vi "Set State.vi"(8 "error in (no error)":errorcluster, 10 "Device State":T1, 11 "Device in":refnum<class "Device.lvclass">) -> (0 "error out":errorcluster, 3 "Device out":refnum<class "Device.lvclass">)   [LabVIEW 2020, in "HAL.lvlib" / "Device.lvclass"]
uses:
  Device.lvclass
  Device State.ctl
  Device.lvclass/Device.ctl
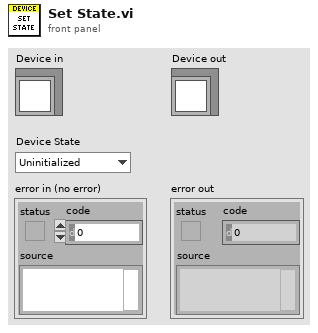
[diagram p1: front panel]
types:
  T1 = typedef "HAL.lvlib/Device.lvclass/Device State.ctl" = enum16{"Uninitialized", "Initialized", "Running", "Error"}
  T2 = typedef "HAL.lvlib/Device.lvclass/Ref Data.ctl" = cluster{"Config Keys":string[], "Config Values":string[], "Cal Expires":timestamp, "Name":string, "Comment":string, "State":T1, "Error":errorcluster}
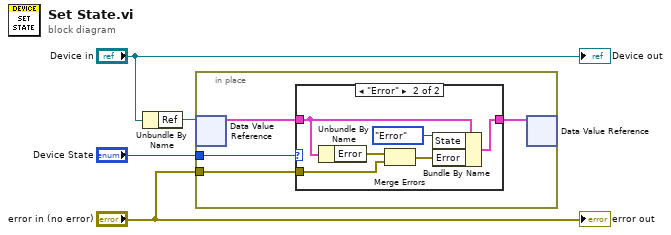
[diagram p0: block diagram]
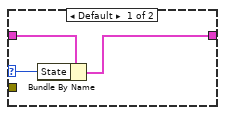
[diagram p2: hidden frame]
diagram:
  n1 = Unbundle By Name("Device in") -> ("Ref"=w4:refnum<data-value>)
  n2 = in-place {
    in-place-border: "Device State" -> [w8]
    in-place-border: "error in (no error)" -> [w7]
    n3 = in-place-dvr #1(w4) -> (w5:T2)  [unwired: 1 out]
    n4 = case shown="\"Error\"" w8 {
      selector: w8 -> [w11 _]
      tunnel: w5 -> [w9 w15]
      tunnel: w7 -> [_ w16]
      tunnel: [w10 w13] -> w6
      frame Default {
        n5 = Bundle By Name(cluster=w9, "State"=w11) -> (w10:T2)
      }
      frame "Error" {
        n6 = Unbundle By Name(w15) -> ("Error"=w17:errorcluster)
        n7 = Merge Errors(w17, w16) -> (w14:errorcluster)
        n8 = Bundle By Name(cluster=w15, "State"=Device_State."Error", "Error"=w14) -> (w13:T2)
      }
    }
    n9 = in-place-dvr #1(w6) -> ()  [unwired: 2 out]
  }
  "error out" <- "error in (no error)"
  "Device out" <- "Device in"
